vi "Gather Test Data - No serial port.vi"(0 "Equipment":T3={"MW100"="COM1", "AG34970"="MW100", "WT210"="A-34972A"}, 5 "Tank Display Ref":refnum<vi>, 11 "error in (no error)":errorcluster) -> (4 "Tc Tree":dbl[](array[numeric]), 6 "Output Data":string[][](array[string]), 8 "POWER":T1, 10 "PowerData":T2={"Voltage (Volts)"=236.2, "Current (Amps)"=17.749, "Power (Watts)"=4192.0, "WattHours (Wh)"=0.0, "TC Tree (AVG)"=0.0, "Flow Rate (GPM)"=0.0, "Gallons (Gal)"=0.0, "RTD Out (Deg F)"=0.0, "TC Down"=0.0}, 15 "error out":errorcluster={"status"=TRUE, "code"=-1073807346, "source"="VISA Read in Gather Test Data.vi"})   [LabVIEW 2014]
uses:
  Type Definitions/PowerElements.ctl
  Type Definitions/EquipReferences.ctl
  Type Definitions/PowerData.ctl
panel:
  out "RTD Out":dbl
  out "Heater Bottom (Lower Element)":dbl
  out "Heater Top (Upper Element)":dbl
  in  "Run Local":bool
  out "Gallons":dbl
  out "Flow Rate":dbl
  out "Tambient":dbl
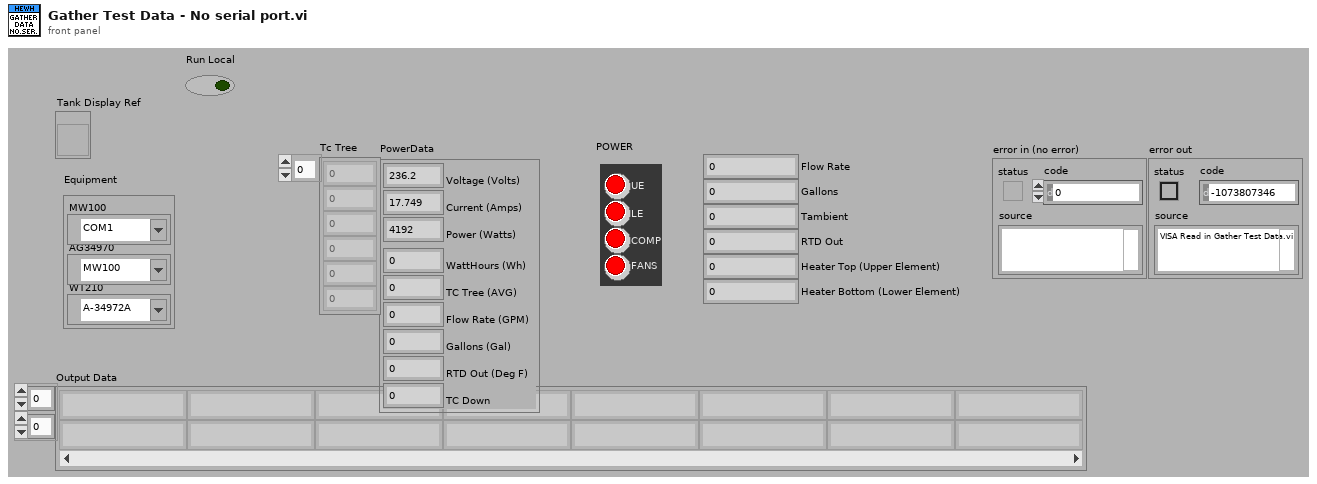
[diagram p1: front panel]
types:
  T1 = typedef "PowerElements.ctl" = cluster{"UE":bool, "LE":bool, "COMP":bool, "FANS":bool}
  T2 = typedef "PowerData.ctl" = cluster{"Voltage (Volts)":dbl, "Current (Amps)":dbl, "Power (Watts)":dbl, "WattHours (Wh)":dbl, "TC Tree (AVG)":dbl, "Flow Rate (GPM)":dbl, "Gallons (Gal)":dbl, "RTD Out (Deg F)":dbl, "TC Down":dbl}
  T3 = typedef "EquipReferences.ctl" = cluster{"MW100":refnum<visa-resource-name>, "AG34970":refnum<visa-resource-name>, "WT210":refnum<visa-resource-name>}
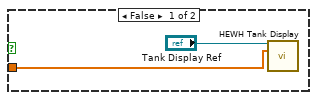
[diagram p2: hidden frame]
diagram:
  w22 = 30.0  # 10V = 300VAC
  # "If the current is in the \nbelow range the compressor\nand fan are on"
  # "Digital Input. If \"ON\" value will be zero"
  # "Digital Input. If \"ON\" value will be zero"
  # "Reference the scan list \nin MW100 Scan for the\nindex locations"
  # "Calculate Pressures"
  # "Let Error Pass if Serial Time Out"
  # "If local, do a local update to the tank graphic.  Otherwise, update the reference."
  # "Samples and Parses all the data for the Fill Test"
  n1 = disable-structure shown="Disabled" {
    frame Disabled {
      w54 = 0.5 ("y")
      # "Look at Heater Top and Bottom Data from MW100"
      n2 = Index Array(index #1=4 ("index"), index #2=5 ("index")) -> (element #1=w56, element #2=w55)  [unwired: 1 in]
      n3 = Less?(x=w56, y=w54) -> ()  [unwired: 1 out]
      n4 = Less?(x=w55, y=w54) -> ()  [unwired: 1 out]
    }
    frame Enabled {
    }
  }
  n5 = Unbundle By Name("Equipment") -> ("MW100"=w48:refnum<visa-resource-name>)
  n6 = call "YKMW100 Receive String-clear buff.vi"("VISA session"=w48, "error in (no error)"="error in (no error)") -> ("dup VISA session"=w47:refnum<visa-resource-name>, "error out"=w46:errorcluster)  [unwired: 11 in, 1 out]
  n7 = call "HEWH Read All MW100 Inputs.vi"("MW100"=w47, "Error In"=w46) -> ("All Data"=w31:dbl[], "error out"=w30:errorcluster)  [unwired: 10 in, 2 out]
  n8 = Unbundle By Name(w30) -> ("status"=w29:bool)
  n9 = call "HEWH Calc Convert Pressure.vi"(8:w31) -> (0:w32)  [unwired: 9 in, 1 out]
  n10 = case shown="True" w29 {
    tunnel: "Equipment" -> [_ w62]
    tunnel: [w59 w61] -> w28
    tunnel: w30 -> [w59 w60]
    frame False {
    }
    frame True {
      n11 = call "HEWH Error Handler.vi"("Equipment"=w62, "error in (no error)"=w60) -> ("Error Out (no error)"=w61:errorcluster)  [unwired: 13 in]
    }
  }
  "error out" <- w28
  n12 = Index Array(array=w31, index #1=20 ("index"), index #2=21 ("index"), index #3=22 ("index"), index #4=8 ("index"), index #5=27 ("index"), index #6=33 ("index"), index #7=35 ("index"), index #8=23 ("index"), index #9=4 ("index"), index #10=5 ("index")) -> (element #1=w44:dbl, element #2=w1:dbl, element #3=w41:dbl, element #4=w36:dbl, element #5=w35:dbl, element #6=w2:dbl, element #7=w3:dbl, element #8=w23:dbl, element #9=w15:dbl, element #10=w14:dbl)
  "Tambient" <- w41
  "Flow Rate" <- w3
  "Gallons" <- w2
  "Heater Top (Upper Element)" <- w15
  "Heater Bottom (Lower Element)" <- w14
  "RTD Out" <- w1
  n13 = Array Subset(array=w31, index=10, length=6) -> (w34:dbl[])
  "Tc Tree" <- w34
  n14 = Multiply(x=w23, y=w22) -> (x*y=w21:dbl)
  n15 = Equal To 0?(x=w15) -> (x = 0?=w13:bool)
  n16 = Equal To 0?(x=w14) -> (x = 0?=w12:bool)
  n17 = Build Array (concatenate)(w34, w44, w1, w41) -> (w50:dbl[])
  n18 = call "HEWH Power Cluster Calcs.vi"("MW100 Data Cluster"=w21, 5:w36, 7:w35, 9:w3, 11:w2, 12:w1) -> ("PowerData"=w11:T2)  [unwired: 8 in, 1 out]
  "PowerData" <- w11
  n19 = case shown="True" "Run Local" {
    tunnel: w50 -> [w64 _]
    frame False {
      n20 = call "HEWH Tank Display.vi"("Local Tank Display"="Tank Display Ref", "T1-T6.Tin,Tout"=w64) -> ()  [unwired: 13 in, 1 out]
    }
    frame True {
    }
  }
  n21 = Unbundle By Name(w11) -> ("Current (Amps)"=w7:dbl)
  n22 = Cluster To Array(cluster=w11) -> (array=w52:dbl[])
  n23 = Less?(x=w7, y=5.0) -> (x < y?=w5:bool)
  n24 = Number To Fractional String(number=w52) -> (F-format string=w51:string[])  [unwired: 3 in]
  n25 = Number To Fractional String(number=w32, precision (6)=i16 2) -> (F-format string=w53:string)  [unwired: 2 in]
  n26 = Greater?(x=w7, y=0.5) -> (0:w6:bool)
  n27 = And(x=w6, y=w5) -> (x .and. y?=w4:bool)
  n28 = call "Parse Heatup Test Data.vi"(10:w51, "MW100 TC Headers"=w53) -> ("Output Data"=→"Output Data":string[][])  [unwired: 9 in]
  n29 = Bundle By Name(cluster=T1 {"UE"=FALSE, "LE"=FALSE, "COMP"=FALSE, "FANS"=FALSE} ("POWER"), "UE"=w13, "LE"=w12, "COMP"=w4, "FANS"=w4) -> (→"POWER":T1)
